vi "Events.vi"(1 "Input":refnum<user-event>, 2 "Event Type":T1, 3 "Action":T2) -> (0 "Output":refnum<user-event>)   [LabVIEW 2013]
uses:
  Functional Globals/Action.ctl
  Event Selector.ctl
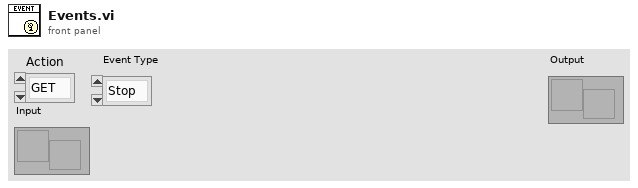
[diagram p1: front panel]
types:
  T1 = typedef "Event Selector.ctl" = enum16{"Stop", "Reload Config"}
  T2 = typedef "Action.ctl" = enum16{"GET", "PUT", "DELETE"}
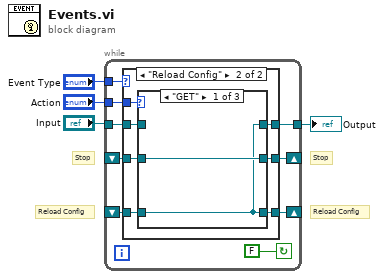
[diagram p0: block diagram]
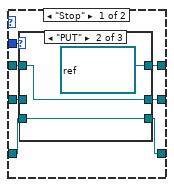
[diagram p2: hidden frame]
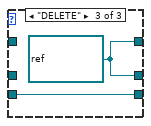
[diagram p4: hidden frame]
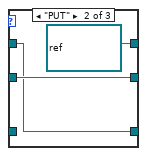
[diagram p5: hidden frame]
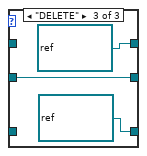
[diagram p6: hidden frame]
diagram:
  # "Reload Config"
  # "Reload Config"
  # "Stop"
  # "Stop"
  n1 = while {
    shift-right: [w10] -> _
    shift-left: _ -> [w9]
    tunnel: "Action" -> [w11]
    tunnel: "Input" -> [w7]
    tunnel: [w8] -> w2
    tunnel: "Event Type" -> [w12]
    shift-right: [w5] -> _
    shift-left: _ -> [w6]
    stop <- FALSE continue-if-true
    n2 = case shown="\"Reload Config\"" w12 {
      tunnel: w11 -> [w20 w31]
      tunnel: [w19 w33] -> w10
      tunnel: w9 -> [w18 w29]
      tunnel: [w17 w34] -> w8
      tunnel: w7 -> [w16 w30]
      tunnel: [w14 w32] -> w5
      tunnel: w6 -> [w15 w28]
      frame "Stop" {
        n3 = case shown="\"PUT\"" w20 {
          tunnel: [w22 w25 w27] -> w19
          tunnel: w18 -> [w22 _ _]
          tunnel: [w22 refnum<user-event> refnum ("Input") w27] -> w17
          tunnel: w16 -> [_ w25 _]
          tunnel: [w21 w23 w26] -> w14
          tunnel: w15 -> [w21 w23 w26]
          frame "GET" {
          }
          frame "PUT" {
          }
          frame "DELETE" {
            w27 = refnum<user-event> refnum ("Input")
          }
        }
      }
      frame "Reload Config" {
        n4 = case shown="\"GET\"" w31 {
          tunnel: [w36 w38 w41] -> w33
          tunnel: w29 -> [w36 w38 w41]
          tunnel: [w35 refnum<user-event> refnum ("Input") refnum<user-event> refnum ("Input")] -> w34
          tunnel: w30 -> [_ w37 _]
          tunnel: [w35 w37 refnum<user-event> refnum ("Input")] -> w32
          tunnel: w28 -> [w35 _ _]
          frame "GET" {
          }
          frame "PUT" {
          }
          frame "DELETE" {
          }
        }
      }
    }
  }
  "Output" <- w2
